vi "Acquire packet.vi"(8 "error in (no error)":errorcluster, 9 "Escape":u8, 10 "Termination":u8, 11 "VISA resource name in":refnum<visa-resource-name>) -> (0 "error out":errorcluster, 2 "Packet":u8[](array[numeric]), 3 "VISA resource name out":refnum<visa-resource-name>)   [LabVIEW 2015, in "Acquisition.lvlib"]
uses:
  Acquisition.lvlib
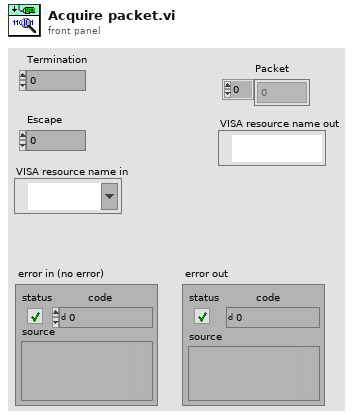
[diagram p1: front panel]
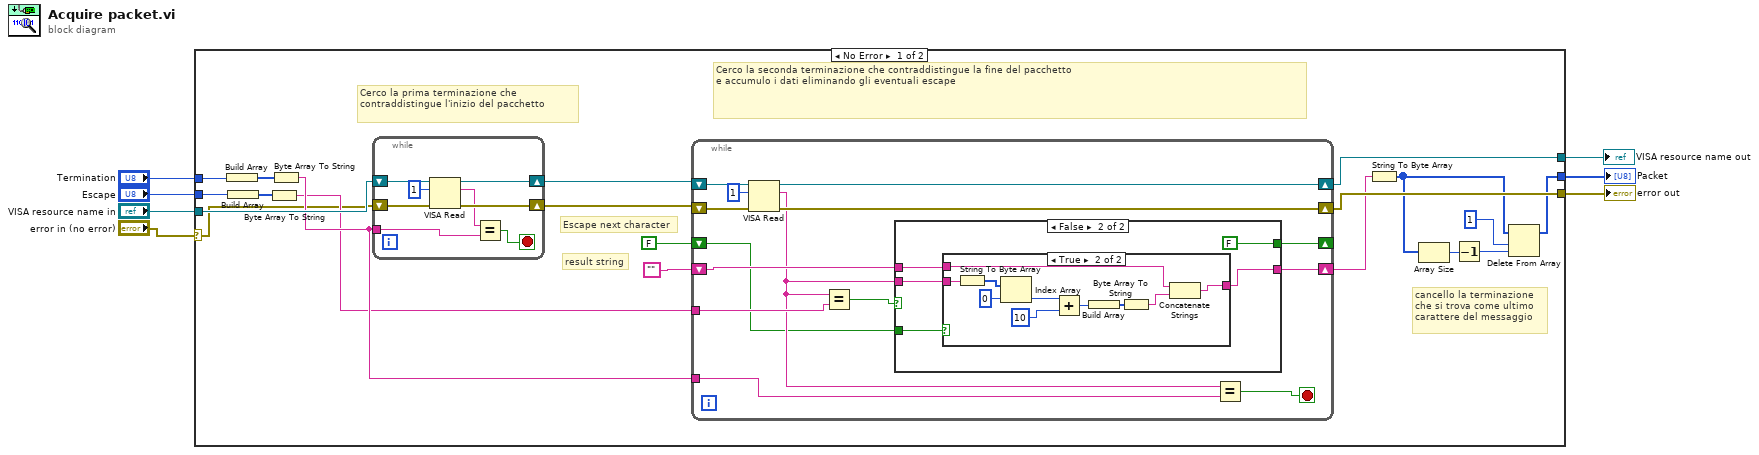
[diagram p0: block diagram]
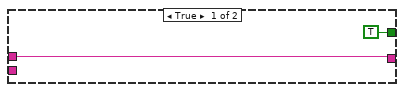
[diagram p2: hidden frame]
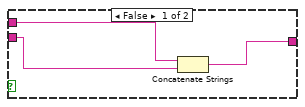
[diagram p3: hidden frame]
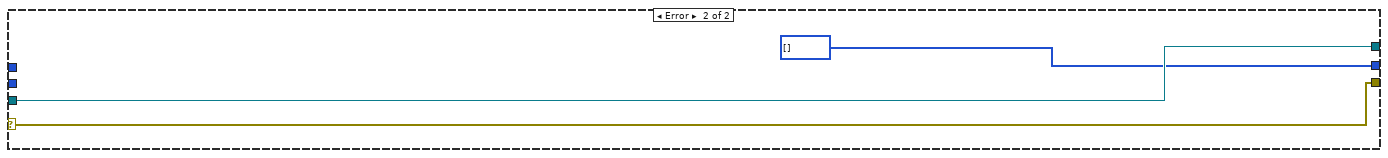
[diagram p4: hidden frame]
diagram:
  n1 = case shown="No Error" "error in (no error)" {
    selector: "error in (no error)" -> [w13 w71]
    tunnel: "Termination" -> [w27 _]
    tunnel: "VISA resource name in" -> [w25 w72]
    tunnel: "Escape" -> [w19 _]
    tunnel: [w16 w71] -> w4
    tunnel: [w12 u8[] [] ("unsigned byte array")] -> w3
    tunnel: [w14 w72] -> w2
    frame No Error {
      # "cancello la terminazione\nche si trova come ultimo\ncarattere del messaggio"
      # "result string"
      # "Escape next character"
      # "Cerco la seconda terminazione che contraddistingue la fine del pacchetto\ne accumulo i dati eliminando gli eventuali escape"
      # "Cerco la prima terminazione che\ncontraddistingue l'inizio del pacchetto"
      n2 = Build Array(w27) -> (w26:u8[])
      n3 = Build Array(w19) -> (w18:u8[])
      n4 = Byte Array To String(unsigned byte array=w18) -> (string=w17:string)
      n5 = Byte Array To String(unsigned byte array=w26) -> (string=w22:string)
      n6 = while {
        shift-right: [w66] -> w23
        shift-left: w25 -> [w69]
        shift-right: [w65] -> w24
        shift-left: w13 -> [w67]
        tunnel: w22 -> [w62]
        stop <- w63 stop-if-true
        n7 = VISA Read(VISA resource name=w69, byte count=u32 1, error in (no error)=w67) -> (VISA resource name out=w66:refnum<visa-resource-name>, read buffer=w64:string, error out=w65:errorcluster)  [unwired: 1 out]
        n8 = Equal?(x=w64, y=w62) -> (x = y?=w63:bool)
      }
      n9 = while {
        shift-right: [w38] -> w14
        shift-left: w23 -> [w41]
        shift-right: [w37] -> w16
        shift-left: w24 -> [w39]
        tunnel: w22 -> [w35]
        shift-right: [w33] -> w15
        shift-left: "" -> [w34]
        shift-right: [w29] -> _
        shift-left: FALSE -> [w28]
        tunnel: w17 -> [w31]
        stop <- w36 stop-if-true
        n10 = VISA Read(VISA resource name=w41, byte count=u32 1, error in (no error)=w39) -> (VISA resource name out=w38:refnum<visa-resource-name>, read buffer=w30:string, error out=w37:errorcluster)  [unwired: 1 out]
        n11 = Equal?(x=w30, y=w31) -> (x = y?=w32:bool)
        n12 = case shown="False" w32 {
          tunnel: w34 -> [w42 w48]
          tunnel: [w42 w47] -> w33
          tunnel: w30 -> [_ w46]
          tunnel: [TRUE FALSE] -> w29
          tunnel: w28 -> [_ w44]
          frame True {
          }
          frame False, Default {
            n13 = case shown="True" w44 {
              tunnel: w48 -> [w51 w60]
              tunnel: [w50 w61] -> w47
              tunnel: w46 -> [w49 w55]
              frame False {
                n14 = Concatenate Strings(w51, w49) -> (w50:string)
              }
              frame True {
                n15 = String To Byte Array(string=w55) -> (unsigned byte array=w54:u8[])
                n16 = Index Array(array=w54, index=0) -> (element=w53:u8)
                n17 = Add(x=w53, y=u8 10) -> (x+y=w57:u8)
                n18 = Build Array(w57) -> (w56:u8[])
                n19 = Byte Array To String(unsigned byte array=w56) -> (string=w58:string)
                n20 = Concatenate Strings(w60, w58) -> (w61:string)
              }
            }
          }
        }
        n21 = Equal?(x=w30, y=w35) -> (x = y?=w36:bool)
      }
      n22 = String To Byte Array(string=w15) -> (unsigned byte array=w11:u8[])
      n23 = Array Size(array=w11) -> (size(s)=w10:i32)
      n24 = Decrement(x=w10) -> (x-1=w9:i32)
      n25 = Delete From Array(array=w11, length=1, index=w9) -> (array with subset deleted=w12:u8[])  [unwired: 1 out]
    }
    frame Error {
    }
  }
  "error out" <- w4
  "Packet" <- w3
  "VISA resource name out" <- w2
